vi "Initialize System.vi"   [LabVIEW 2014, in "NI_EP_Power Quality.lvlib"]
doc: "Sets the basic configuration of the electrical power system based on different line and bus configurations. You must manually select the polymorphic instance you want to use."
uses:
  <vilib>/addons/Electrical Power/PQ/NI_EP_Power Quality.lvlib
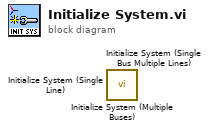
[diagram p0: block diagram]
diagram:
  n1 = call <vilib>:"Initialize System (Multiple Buses).vi"() -> ()  [unwired: 13 in, 3 out]
  n2 = call <vilib>:"Initialize System (Single Bus Multiple Lines).vi"() -> ()  [unwired: 13 in, 3 out]
  n3 = call <vilib>:"Initialize System (Single Line).vi"() -> ()  [unwired: 13 in, 3 out]
